vi "AB_Is_Destination_Present.vi"(8 "error in (no error)":errorcluster, 10 "destination label":string, 11 "destinations":refnum<class "AB_Destination.lvclass">[](array[class])) -> (0 "error out":errorcluster, 2 "index":i32, 3 "destination present?":bool)   [LabVIEW 2020]
uses:
  <vilib>/AppBuilder/AB_Classes/Destination/AB_Destination.lvclass
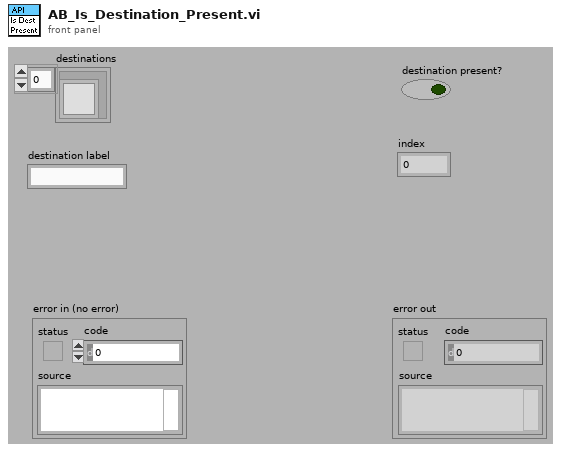
[diagram p1: front panel]
types:
  T1 = typedef "AB_Destination.ctl" = cluster{"destName":string, "path":path, "libraryName":string, "preserveHierarchy":bool, "eng_inBuild":bool, "eng_libraryReference":refnum<vi>, "eng_restictAddToNewLibrary":bool}
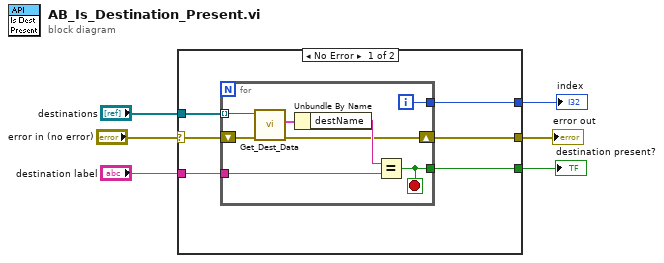
[diagram p0: block diagram]
diagram:
  n1 = case shown="No Error" "error in (no error)" {
    selector: "error in (no error)" -> [w8 w21]
    tunnel: [w12 _] -> w6
    tunnel: [w11 _] -> w5
    tunnel: "destination label" -> [w10 _]
    tunnel: "destinations" -> [w9 _]
    tunnel: [w7 w21] -> w1
    frame No Error {
      n2 = for {
        tunnel: w9 -> [w20] mode=indexing
        tunnel: w10 -> [w18]
        tunnel: [w17] -> w11
        tunnel: [w16] -> w12
        shift-right: [w13] -> w7
        shift-left: w8 -> [w14]
        i -> [w16]
        stop <- w17 stop-if-true
        n3 = call <vilib>:"Get_Dest_Data.vi"("error in (no error)"=w14, "Class in"=w20) -> ("error out"=w13:errorcluster, "destName"=w19:T1)  [unwired: 8 out]
        n4 = Unbundle By Name(w19) -> ("destName"=w15:string)
        n5 = Equal?(x=w15, y=w18) -> (x = y?=w17:bool)
      }
    }
    frame Error {
    }
  }
  "index" <- w6
  "destination present?" <- w5
  "error out" <- w1
